vi "Validate Peripheral.vi"(8 "error in (no error)":errorcluster, 9 "EVI (\"\")":string, 10 "Peripheral Name":string, 11 "FPGA Personality File Path":path) -> (0 "error out":errorcluster, 2 "Supported?":bool, 3 "Duplicated FPGA Personality File Path":path)   [LabVIEW 2021, in "Personality.lvlib"]
doc: "Checks if the peripheral/EVI is supported by the specified FPGA persoanlity file."
uses:
  <vilib>/myRIO/Common/FPGA Personality Framework/Personality.lvlib
  <vilib>/xml/Load XML File.vi
  <vilib>/xml/Close Reference(Node).vi
  <vilib>/xml/NI_XML.lvlib
  <resource>/objmgr/DOMUserDefRef.rc
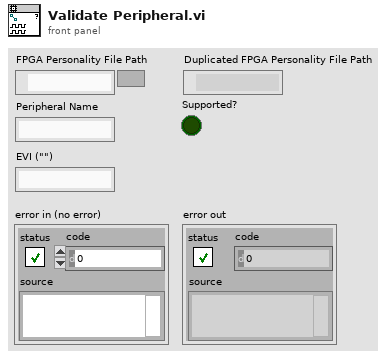
[diagram p1: front panel]
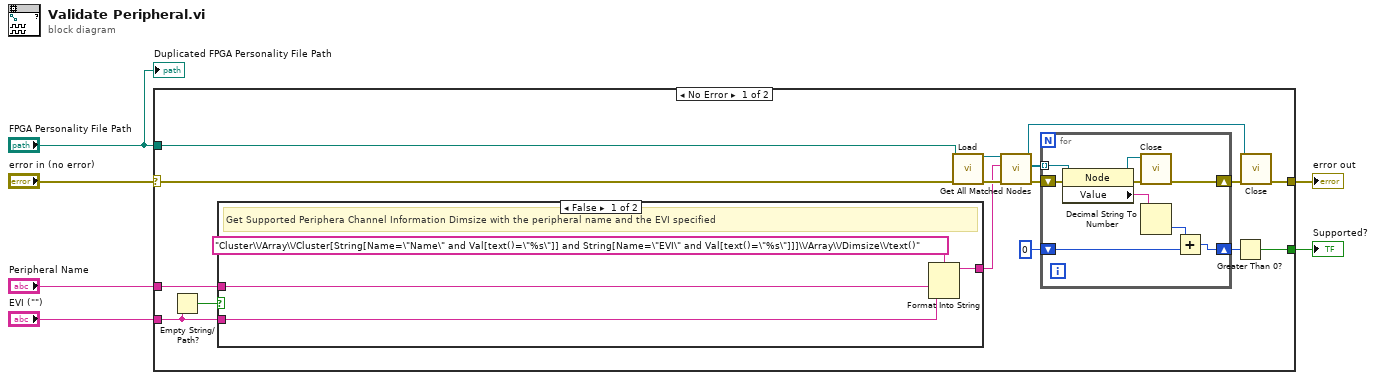
[diagram p0: block diagram]
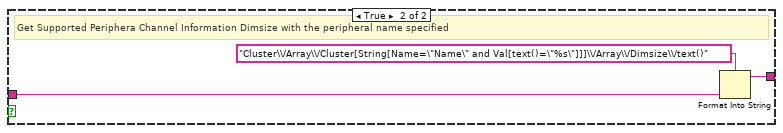
[diagram p2: hidden frame]
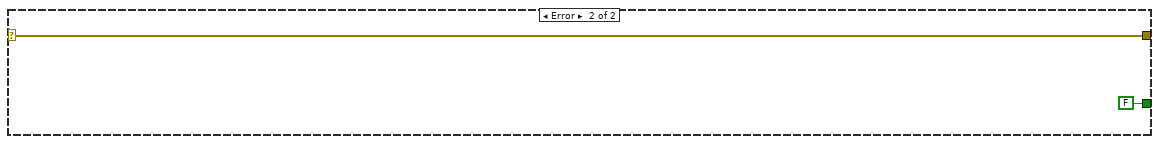
[diagram p3: hidden frame]
diagram:
  n1 = case shown="No Error" "error in (no error)" {
    selector: "error in (no error)" -> [w22 w40]
    tunnel: [w21 w40] -> w5
    tunnel: "FPGA Personality File Path" -> [w20 _]
    tunnel: "Peripheral Name" -> [w16 _]
    tunnel: "EVI (\"\")" -> [w15 _]
    tunnel: [w11 FALSE] -> w1
    frame No Error {
      n2 = Empty String/Path?(string/path=w15) -> (empty?=w17:bool)
      n3 = case shown="False" w17 {
        tunnel: w16 -> [w34 w37]
        tunnel: [w33 w36] -> w14
        tunnel: w15 -> [w32 _]
        frame False {
          # "Get Supported Periphera Channel Information Dimsize with the peripheral name and the EVI specified"
          n4 = Format Into String(format string="Cluster\\/Array\\/Cluster[String[Name=\"Name\" and Val[text()=\"%s\"]] and String[Name=\"EVI\" and Val[text()=\"%s\"]]]\\/Array\\/Dimsize\\/text()", w34, w32) -> (resulting string=w33:string)  [unwired: 2 in, 1 out]
        }
        frame True {
          # "Get Supported Periphera Channel Information Dimsize with the peripheral name specified"
          n5 = Format Into String(format string="Cluster\\/Array\\/Cluster[String[Name=\"Name\" and Val[text()=\"%s\"]]]\\/Array\\/Dimsize\\/text()", w37) -> (resulting string=w36:string)  [unwired: 2 in, 1 out]
        }
      }
      n6 = call-poly <vilib>:"Load.vi"("path to XML document"=w20, "error in (no error)"=w22) -> ("DOM document out"=w19:refnum<k20>, "error out"=w18:errorcluster)  [unwired: 11 in, 1 out]
      n7 = call <vilib>:"Get All Matched Nodes.vi"("error in (no error)"=w18, "XPath expression"=w14, "node in"=w19) -> ("error out"=w9:errorcluster, "node result array"=w13:refnum<k20>[], "node out"=w7:refnum<k20>)  [unwired: 6 in]
      n8 = for {
        tunnel: w13 -> [w31] mode=indexing
        shift-right: [w27] -> w10
        shift-left: w9 -> [w28]
        shift-right: [w24] -> w12
        shift-left: 0 -> [w23]
        n9 = property class="Node"(reference=w31, error in=w28) -> (reference out=w26:refnum<k20>, error out=w29:errorcluster, "Value"=w30:string)
        n10 = call-poly <vilib>:"Close.vi"("error in (no error)"=w29, "node"=w26) -> ("error out"=w27:errorcluster)  [unwired: 7 in]
        n11 = Decimal String To Number(string=w30) -> (number=w25:i32)  [unwired: 2 in, 1 out]
        n12 = Add(x=w25, y=w23) -> (x+y=w24:i32)
      }
      n13 = Greater Than 0?(x=w12) -> (x > 0?=w11:bool)
      n14 = call-poly <vilib>:"Close.vi"("error in (no error)"=w10, "node"=w7) -> ("error out"=w21:errorcluster)  [unwired: 7 in]
    }
    frame Error {
    }
  }
  "error out" <- w5
  "Supported?" <- w1
  "Duplicated FPGA Personality File Path" <- "FPGA Personality File Path"
